vi "LJUD UE9RAW ControlConfig.vi"(5 "Digital Defaults [1]":T2, 6 "DAC Defaults [2]":cluster{"DAC0":u16, "DAC1":u16, "Enabled":bool}, 7 "Comm Settings":T3={"Open LabJack "=TRUE, "Use USB"=TRUE, "IP Address"="192.168.1.209", "PortA"=52360, "PortB"=0}, 8 "error in (no error)":errorcluster, 9 "Power Level [0]":u8, 10 "WriteMask":u8, 11 "Handle In":i32) -> (0 "error out":errorcluster, 1 "Defaults Read":T1, 2 "Flash Mode":bool, 3 "Handle Out":i32, 4 "Params":T4 {"Control Bootloader Version" format="%.2f"; "Control Firmware Version" format="%.2f"})   [LabVIEW 2021]
panel:
  out "Read Array":u8[](array[numeric]) format="%.0x"
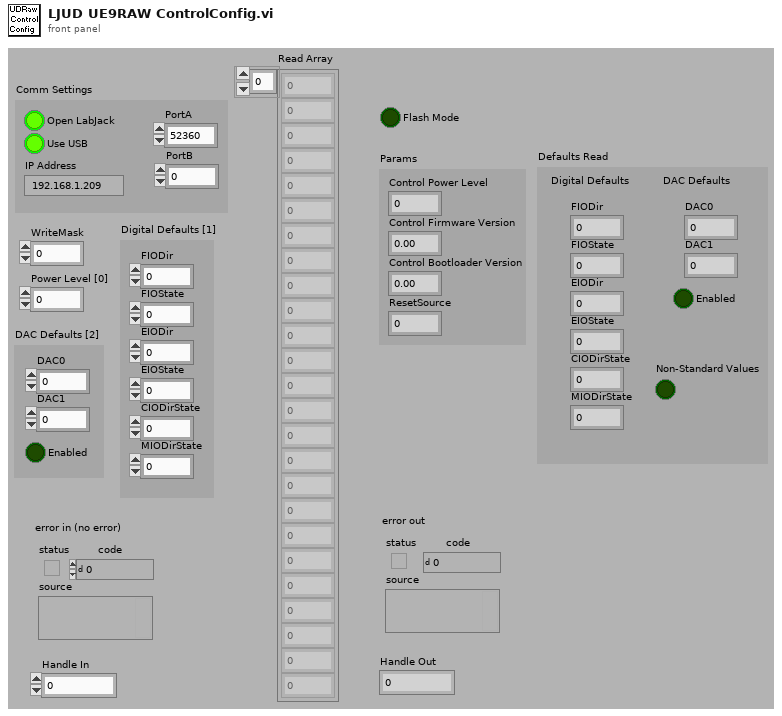
[diagram p1: front panel]
types:
  T1 = cluster{"Digital Defaults":cluster{"FIODir":u8, "FIOState":u8, "EIODir":u8, "EIOState":u8, "CIODirState":u8, "MIODirState":u8}, "DAC Defaults":cluster{"DAC0":u16, "DAC1":u16, "Enabled":bool}, "Non-Standard Values":bool}
  T2 = cluster{"FIODir":u8, "FIOState":u8, "EIODir":u8, "EIOState":u8, "CIODirState":u8, "MIODirState":u8}
  T3 = cluster{"Open LabJack ":bool, "Use USB":bool, "IP Address":string, "PortA":u16, "PortB":u16}
  T4 = cluster{"Control Firmware Version":dbl, "Control Bootloader Version":dbl, "Control Power Level":u8, "ResetSource":u8}
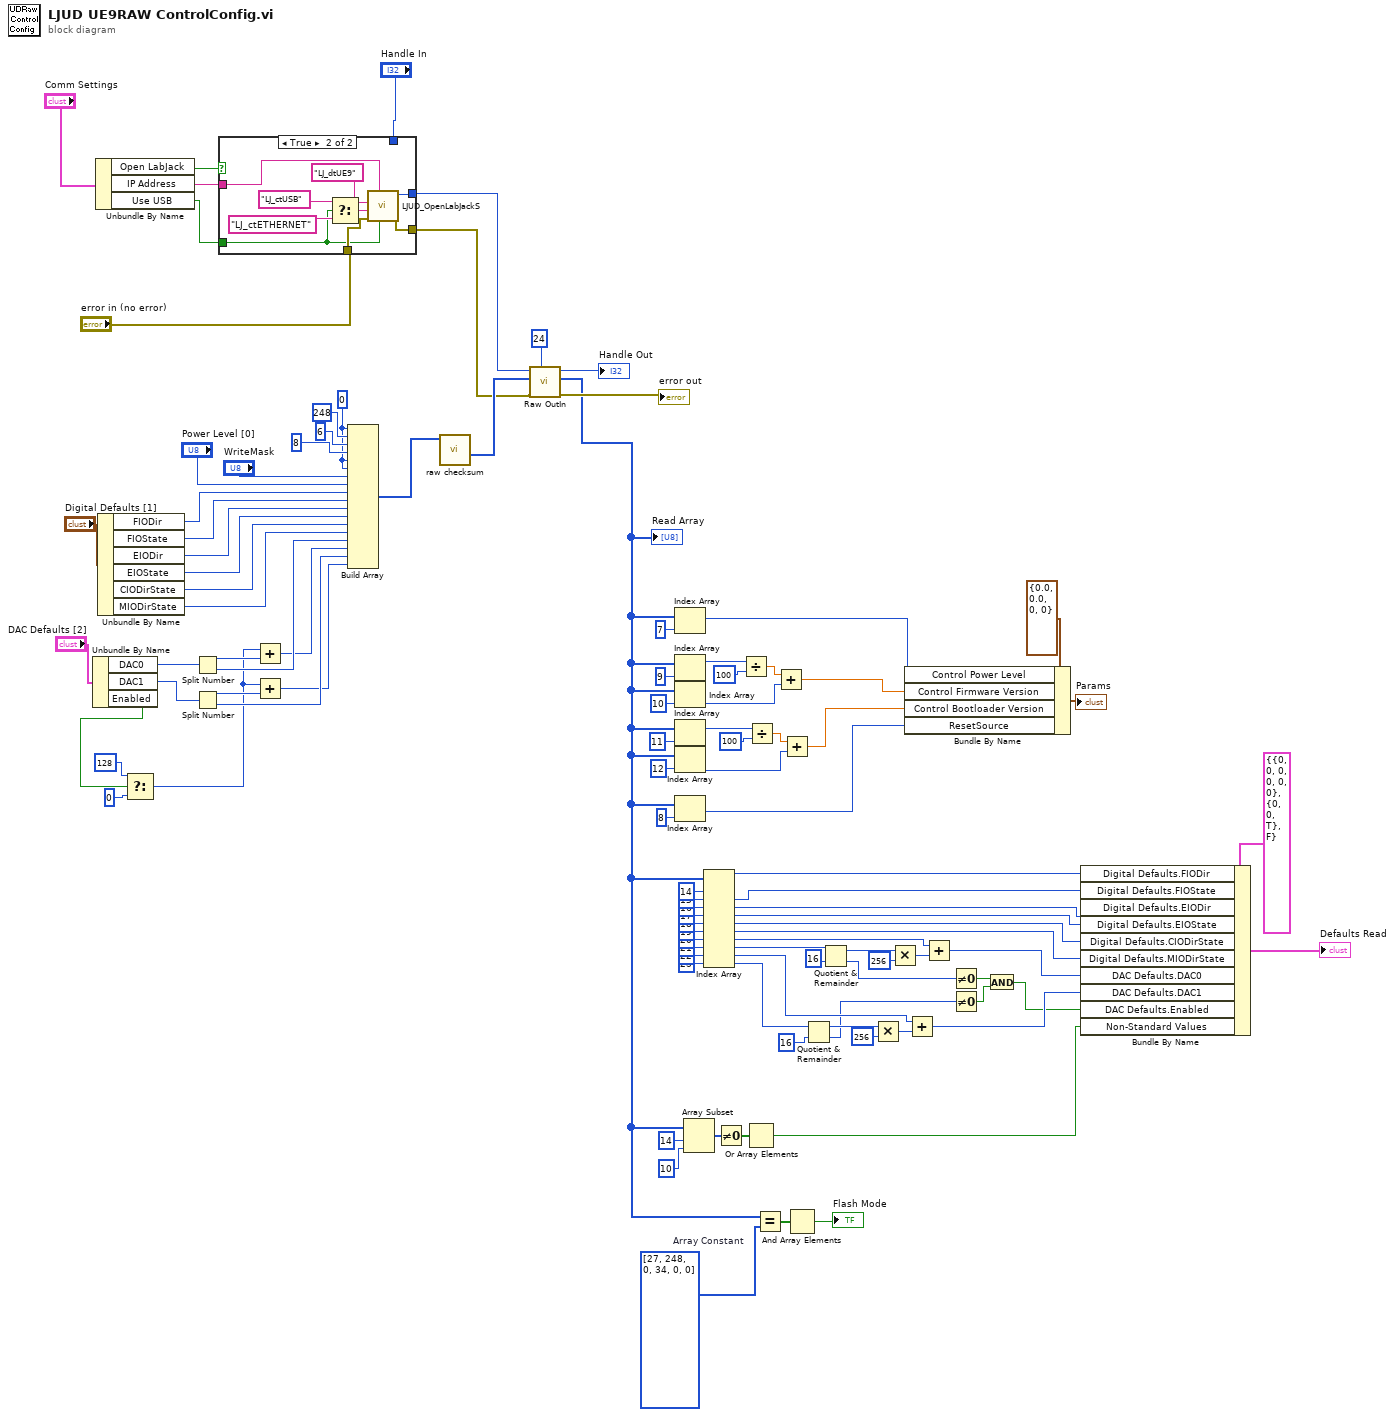
[diagram p0: block diagram]
diagram:
  w83 = u8[] [27, 248, 0, 34, 0, 0]  # Array Constant
  w52 = u8 0 ("Input Element")
  n1 = Unbundle By Name("DAC Defaults [2]") -> ("DAC0"=w59:u16, "DAC1"=w58:u16, "Enabled"=w60:bool)
  n2 = Unbundle By Name("Comm Settings") -> ("Open LabJack"=w1:bool, "IP Address"=w2:string, "Use USB"=w3:bool)
  n3 = Unbundle By Name("Digital Defaults [1]") -> ("FIODir"=w71:u8, "FIOState"=w70:u8, "EIODir"=w69:u8, "EIOState"=w68:u8, "CIODirState"=w67:u8, "MIODirState"=w66:u8)
  n4 = Select(t=u8 128 ("x"), s=w60, f=u8 0 ("x")) -> (s? t:f=w8:u8)
  n5 = Split Number(x=w59) -> (hi(x)=w62:u8, lo(x)=w57:u8)
  n6 = Split Number(x=w58) -> (hi(x)=w61:u8, lo(x)=w55:u8)
  n7 = case shown="True" w1 {
    tunnel: w2 -> [_ w110]
    tunnel: "error in (no error)" -> [w107 w114]
    tunnel: [w107 w113] -> w6
    tunnel: [w106 w111] -> w7
    tunnel: w3 -> [_ w112]
    tunnel: "Handle In" -> [w106 _]
    frame False {
    }
    frame True {
      n8 = Select(t="LJ_ctUSB" ("ConnectionType"), s=w112, f="LJ_ctETHERNET" ("ConnectionType")) -> (s? t:f=w108:string)
      n9 = call "LJUD_OpenLabJackS.vi"("FirstFound"=w112, "Address"=w110, "error in"=w114, "ConnectionType"=w108, "DeviceType"="LJ_dtUE9") -> ("error out"=w113:errorcluster, "Handle"=w111:i32)  [unwired: 4 in, 1 out]
    }
  }
  n10 = Add(x=w8, y=w62) -> (x+y=w56:u8)
  n11 = Add(x=w8, y=w61) -> (x+y=w54:u8)
  n12 = Build Array(w52, u8 248 ("Input Element"), u8 6 ("Input Element"), u8 8 ("Input Element"), w52, w52, "WriteMask", "Power Level [0]", w71, w70, w69, w68, w67, w66, w57, w56, w55, w54) -> (w88:u8[])
  n13 = call "raw checksum.vi"("Array"=w88) -> ("Array Output"=w77:u8[])  [unwired: 3 in, 7 out]
  n14 = call "Raw OutIn.vi"("# of bytes to read in"=24 ("# of bytes to read"), "error in"=w6, "Raw Out"=w77, "Handle In"=w7) -> ("error out"=→"error out":errorcluster, "Raw In"=w49:u8[], "Handle Out"=→"Handle Out":i32)  [unwired: 4 in, 1 out]
  "Read Array" <- w49
  n15 = Index Array(array=w49, index=7 ("Index")) -> (element=w87:u8)
  n16 = Index Array(array=w49, index=9 ("Index")) -> (element=w96:u8)
  n17 = Index Array(array=w49, index=10 ("Index")) -> (element=w93:u8)
  n18 = Index Array(array=w49, index=11 ("Index")) -> (element=w90:u8)
  n19 = Index Array(array=w49, index=12 ("Index")) -> (element=w89:u8)
  n20 = Index Array(array=w49, index=8 ("Index")) -> (element=w84:u8)
  n21 = Array Subset(array=w49, index=14 ("Array Index"), length=10 ("Array Length")) -> (w46:u8[])
  n22 = Index Array(array=w49, index #1=14 ("Index"), index #2=15 ("Index"), index #3=16 ("Index"), index #4=17 ("Index"), index #5=18 ("Index"), index #6=19 ("Index"), index #7=20 ("Index"), index #8=21 ("Index"), index #9=22 ("Index"), index #10=23 ("Index")) -> (element #1=w35:u8, element #2=w34:u8, element #3=w33:u8, element #4=w32:u8, element #5=w31:u8, element #6=w30:u8, element #7=w24:u8, element #8=w29:u8, element #9=w18:u8, element #10=w17:u8)
  n23 = Not Equal To 0?(x=w46) -> (x != 0?=w45:bool[])
  n24 = Divide(x=w96, y=u8 100) -> (x/y=w94:dbl)
  n25 = Or Array Elements(Boolean array=w45) -> (logical OR=w44:bool)
  n26 = Divide(x=w90, y=u8 100) -> (x/y=w92:dbl)
  n27 = Equal?(x=w49, y=w83) -> (x = y?=w82:bool[])
  n28 = Add(x=w94, y=w93) -> (x+y=w86:dbl)
  n29 = Add(x=w92, y=w89) -> (x+y=w85:dbl)
  n30 = And Array Elements(Boolean array=w82) -> (logical AND=→"Flash Mode":bool)
  n31 = Quotient & Remainder(x=w17, y=u16 16) -> (x-y*floor(x/y)=w20:u16, floor(x/y)=w13:u16)
  n32 = Quotient & Remainder(x=w29, y=u16 16) -> (x-y*floor(x/y)=w27:u16, floor(x/y)=w14:u16)
  n33 = Multiply(x=w20, y=u16 256) -> (x*y=w22:u16)
  n34 = Multiply(x=w27, y=u16 256) -> (x*y=w25:u16)
  n35 = Bundle By Name(cluster=T4 {"Control Firmware Version"=0.0, "Control Bootloader Version"=0.0, "Control Power Level"=0, "ResetSource"=0} ("Params"), "Control Power Level"=w87, "Control Firmware Version"=w86, "Control Bootloader Version"=w85, "ResetSource"=w84) -> (→"Params":T4)
  n36 = Add(x=w18, y=w22) -> (x+y=w16:u16)
  n37 = Add(x=w24, y=w25) -> (x+y=w23:u16)
  n38 = Not Equal To 0?(x=w14) -> (x != 0?=w15:bool)
  n39 = Not Equal To 0?(x=w13) -> (x != 0?=w12:bool)
  n40 = And(x=w15, y=w12) -> (x .and. y?=w11:bool)
  n41 = Bundle By Name(cluster=T1 {"Digital Defaults"={"FIODir"=0, "FIOState"=0, "EIODir"=0, "EIOState"=0, "CIODirState"=0, "MIODirState"=0}, "DAC Defaults"={"DAC0"=0, "DAC1"=0, "Enabled"=TRUE}, "Non-Standard Values"=FALSE} ("Defaults Read"), "Digital Defaults.FIODir"=w35, "Digital Defaults.FIOState"=w34, "Digital Defaults.EIODir"=w33, "Digital Defaults.EIOState"=w32, "Digital Defaults.CIODirState"=w31, "Digital Defaults.MIODirState"=w30, "DAC Defaults.DAC0"=w23, "DAC Defaults.DAC1"=w16, "DAC Defaults.Enabled"=w11, "Non-Standard Values"=w44) -> (→"Defaults Read":T1)
